vi "Get Gyro Sensor.vi"() -> (2 "Robot Field Orientation (deg)":dbl, 3 "ADIS Gyro Values":T1 {"IMU Data Out"."X Accel (g)" format="%#_3g"; "IMU Data Out"."Y Accel (g)" format="%#_3g"; "IMU Data Out"."Z Accel (g)" format="%#_3g"})   [LabVIEW 2018]
uses:
  ADIS Gyro Values.ctl
  <vilib>/Rock Robotics/Network Tables/NT Write Number.vi
  gyro sensor adis/ADIS16448 IMU/ADIS16448_IMU.lvlib
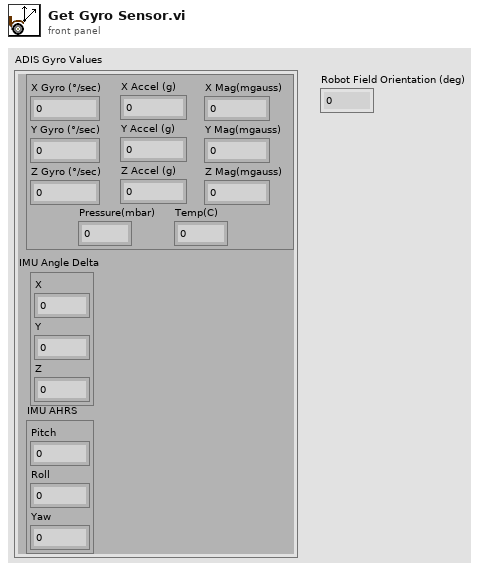
[diagram p1: front panel]
types:
  T1 = typedef "ADIS Gyro Values.ctl" = cluster{"IMU Data Out":cluster{"X Gyro (°/sec)":dbl, "Y Gyro (°/sec)":dbl, "Z Gyro (°/sec)":dbl, "X Accel (g)":dbl, "Y Accel (g)":dbl, "Z Accel (g)":dbl, "X Mag(mgauss)":dbl, "Y Mag(mgauss)":dbl, "Z Mag(mgauss)":dbl, "Pressure(mbar)":dbl, "Temp(C)":dbl}, "IMU Angle Delta":cluster{"X":dbl, "Y":dbl, "Z":dbl}, "IMU AHRS":cluster{"Pitch":dbl, "Roll":dbl, "Yaw":dbl}}
  T2 = typedef "ADIS16448_IMU.lvlib/ADI_IMU_ADIS16448_IMUDevRef.ctl" = cluster{"DevStatus":errorcluster, "Handle":i32, "SPI Bus":T3, "Device Found":bool, "Device Ready":bool, "Yaw Axis":enum16{"X", "Y", "Z"}, "AHRS Algorithm":enum16{"Complementary", "Madgwick"}, "Serial":u16, "Lot ID 2":u16, "Lot ID 1":u16, "Bytes Per Sample":u16, "Calibrate On Open?":bool}
  T3 = typedef "spi_bus.ctl" = enum16{"SPI On-Board, CS0", "SPI On-Board, CS1", "SPI On-Board, CS2", "SPI On-Board, CS3", "SPI MXP", "Invalid"}
  T4 = cluster{"X Gyro":dbl, "Y Gyro":dbl, "Z Gyro":dbl, "X Accel":dbl, "Y Accel":dbl, "Z Accel":dbl, "X Mag":dbl, "Y Mag":dbl, "Z Mag":dbl, "Pressure":dbl, "Temp":dbl}
  T5 = cluster{"X Angle":dbl, "Y Angle":dbl, "Z Angle":dbl}
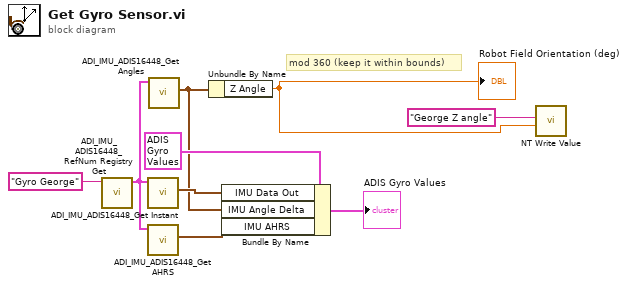
[diagram p0: block diagram]
diagram:
  # "mod 360 (keep it within bounds)"
  n1 = call "ADI_IMU_ADIS16448_RefNum Registry Get.vi"("refnum name"="Gyro George") -> ("ADI IMU DevRef"=w8:T2)  [unwired: 9 in, 1 out]
  n2 = call "ADI_IMU_ADIS16448_Get Instant.vi"("ADI IMU DevRef"=w8) -> ("IMU Data Out"=w5:T4)  [unwired: 7 in, 3 out]
  n3 = call "ADI_IMU_ADIS16448_Get AHRS.vi"("ADI IMU DevRef"=w8) -> ("IMU AHRS Out"=w4:cluster{"Pitch":dbl, "Roll":dbl, "Yaw":dbl})  [unwired: 7 in, 3 out]
  n4 = call "ADI_IMU_ADIS16448_Get Angles.vi"("ADI IMU DevRef"=w8) -> ("IMU Angles Out"=w3:T5)  [unwired: 7 in, 3 out]
  n5 = Unbundle By Name(w3) -> ("Z Angle"=w1:dbl)
  "Robot Field Orientation (deg)" <- w1
  n6 = Bundle By Name(cluster=T1 {"IMU Data Out"={"X Gyro (°/sec)"=0.0, "Y Gyro (°/sec)"=0.0, "Z Gyro (°/sec)"=0.0, "X Accel (g)"=0.0, "Y Accel (g)"=0.0, "Z Accel (g)"=0.0, "X Mag(mgauss)"=0.0, "Y Mag(mgauss)"=0.0, "Z Mag(mgauss)"=0.0, "Pressure(mbar)"=0.0, "Temp(C)"=0.0}, "IMU Angle Delta"={"X"=0.0, "Y"=0.0, "Z"=0.0}, "IMU AHRS"={"Pitch"=0.0, "Roll"=0.0, "Yaw"=0.0}} ("ADIS Gyro Values"), "IMU Data Out"=w5, "IMU Angle Delta"=w3, "IMU AHRS"=w4) -> (→"ADIS Gyro Values":T1)
  n7 = call-poly <vilib>:"NT Write Value.vi"("Numeric"=w1, "Name"="George Z angle") -> ()  [unwired: 9 in, 1 out]
